vi "Create Channel Task Manual.vi"(8 "error in (no error)":errorcluster, 9 "Waveform Generation":T1(array[cluster]), 10 "SQL query":string="SELECT max(MaximumVoltage),max(MinimumVoltage), max(TerminalConfiguration),max(SampleRate) FROM ltt.daq_configuration \nWhere ChannelType='Analog_Output' and Enabled=1;", 11 "AO in":refnum<class "AO.lvclass">) -> (0 "error out":errorcluster, 3 "AO out":refnum<class "AO.lvclass">)   [LabVIEW 2023, in "HardwareAbstractionLayer_LVOOP.lvlib" / "AO.lvclass"]
uses:
  AO.lvclass
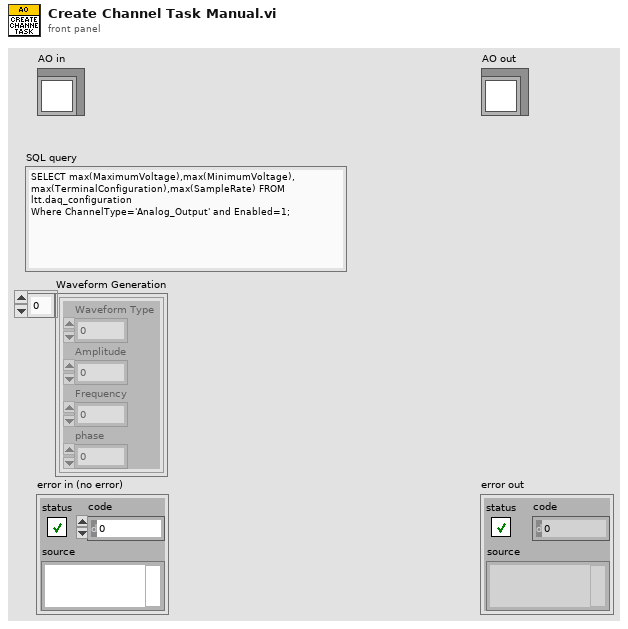
[diagram p1: front panel]
types:
  T1 = cluster{"Waveform Type":u16, "Amplitude":dbl, "Frequency":dbl, "phase":dbl}[]
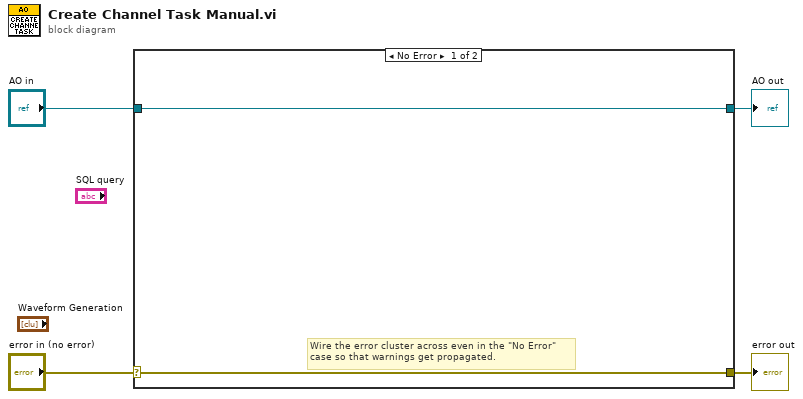
[diagram p0: block diagram]
diagram:
  n1 = case shown="No Error" "error in (no error)" {
    selector: "error in (no error)" -> [w5 w8]
    tunnel: [w5 w8] -> w3
    tunnel: [w6 w7] -> w1
    tunnel: "AO in" -> [w6 w7]
    frame No Error {
      # "Wire the error cluster across even in the \"No Error\"\ncase so that warnings get propagated."
    }
    frame Error {
    }
  }
  "error out" <- w3
  "AO out" <- w1
